vi "Enqueue UI handling loop data.vi"(6 "Next State":T1, 7 "Priority Message? (T)":bool=TRUE, 8 "error in (no error)":errorcluster, 9 "Start/Stop":T2, 10 "Message":string, 11 "Queue in":refnum<queue>) -> (0 "error out":errorcluster, 3 "Queue out":refnum<queue>)   [LabVIEW 2017]
uses:
  Typedefs/Start-Stop Enum.ctl
  Message Queue/Typedefs/Message Cluster.ctl
  Typedefs/Top level VI states.ctl
  Typedefs/Next state queue data.ctl
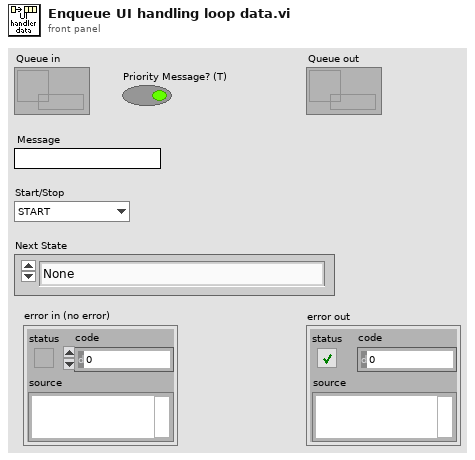
[diagram p1: front panel]
types:
  T1 = typedef "Top level VI states.ctl" = enum16{"None", "Initialise UI", "<STACK PROTOCOL STATES>", "AOL Zstack-START", "AOL Zstack-STOP", "Motor Zstack-START", "Motor Zstack-STOP", "<ACQUISITION PROTOCOL STATES> ", "Functional Acquisition-START", "Functional Acquisition-STOP", "Single Plane Acquisition-START", "Single Plane Acquisition-STOP", "Volume Acquisition-START", "Volume Acquisition-STOP", "<LIVE IMAGING PROTOCOL STATES>", "Live Imaging-START", "Live Imaging-STOP", "Live Plane Imaging-START", "Live Plane Imaging-STOP", "Live Volume Imaging-START", "Live Volume Imaging-STOP", "<MOVEMENT CORRECTION PROTOCOL STATES>", "Background MovCor-START", "Background MovCor-STOP", "EXIT"}
  T2 = typedef "Start-Stop Enum.ctl" = enum16{"START", "STOP"}
  T3 = typedef "Next state queue data.ctl" = cluster{"Start/Stop":T2, "State":T1}
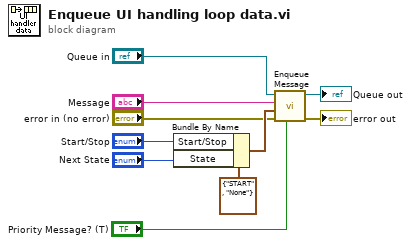
[diagram p0: block diagram]
diagram:
  n1 = Bundle By Name(cluster=T3 {"Start/Stop"=enum."START", "State"=enum."None"}, "Start/Stop"="Start/Stop", "State"="Next State") -> (w9:T3)
  n2 = call "Enqueue Message.vi"("Priority Message? (F)"="Priority Message? (T)", "error in (no error)"="error in (no error)", "Message Data"=w9, "Message"="Message", "Queue"="Queue in") -> ("error out"=→"error out":errorcluster, "Queue out"=→"Queue out":refnum<queue>)  [unwired: 5 in]
